vi "Arm State Machine.vi"(1 "Delta Angle":dbl, 2 "Shoulder Control":bool, 3 "Forearm Control":bool, 4 "State":i32) -> (0 "Next State":i32)   [LabVIEW 2017]
uses:
  Robot Global Data.vi
panel:
  in  "Controller Multiplier":dbl=0.5
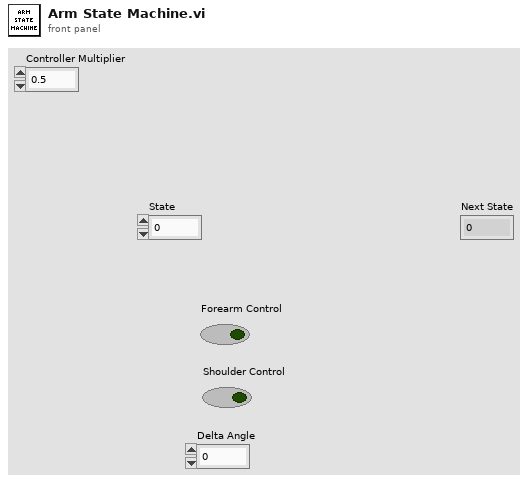
[diagram p1: front panel]
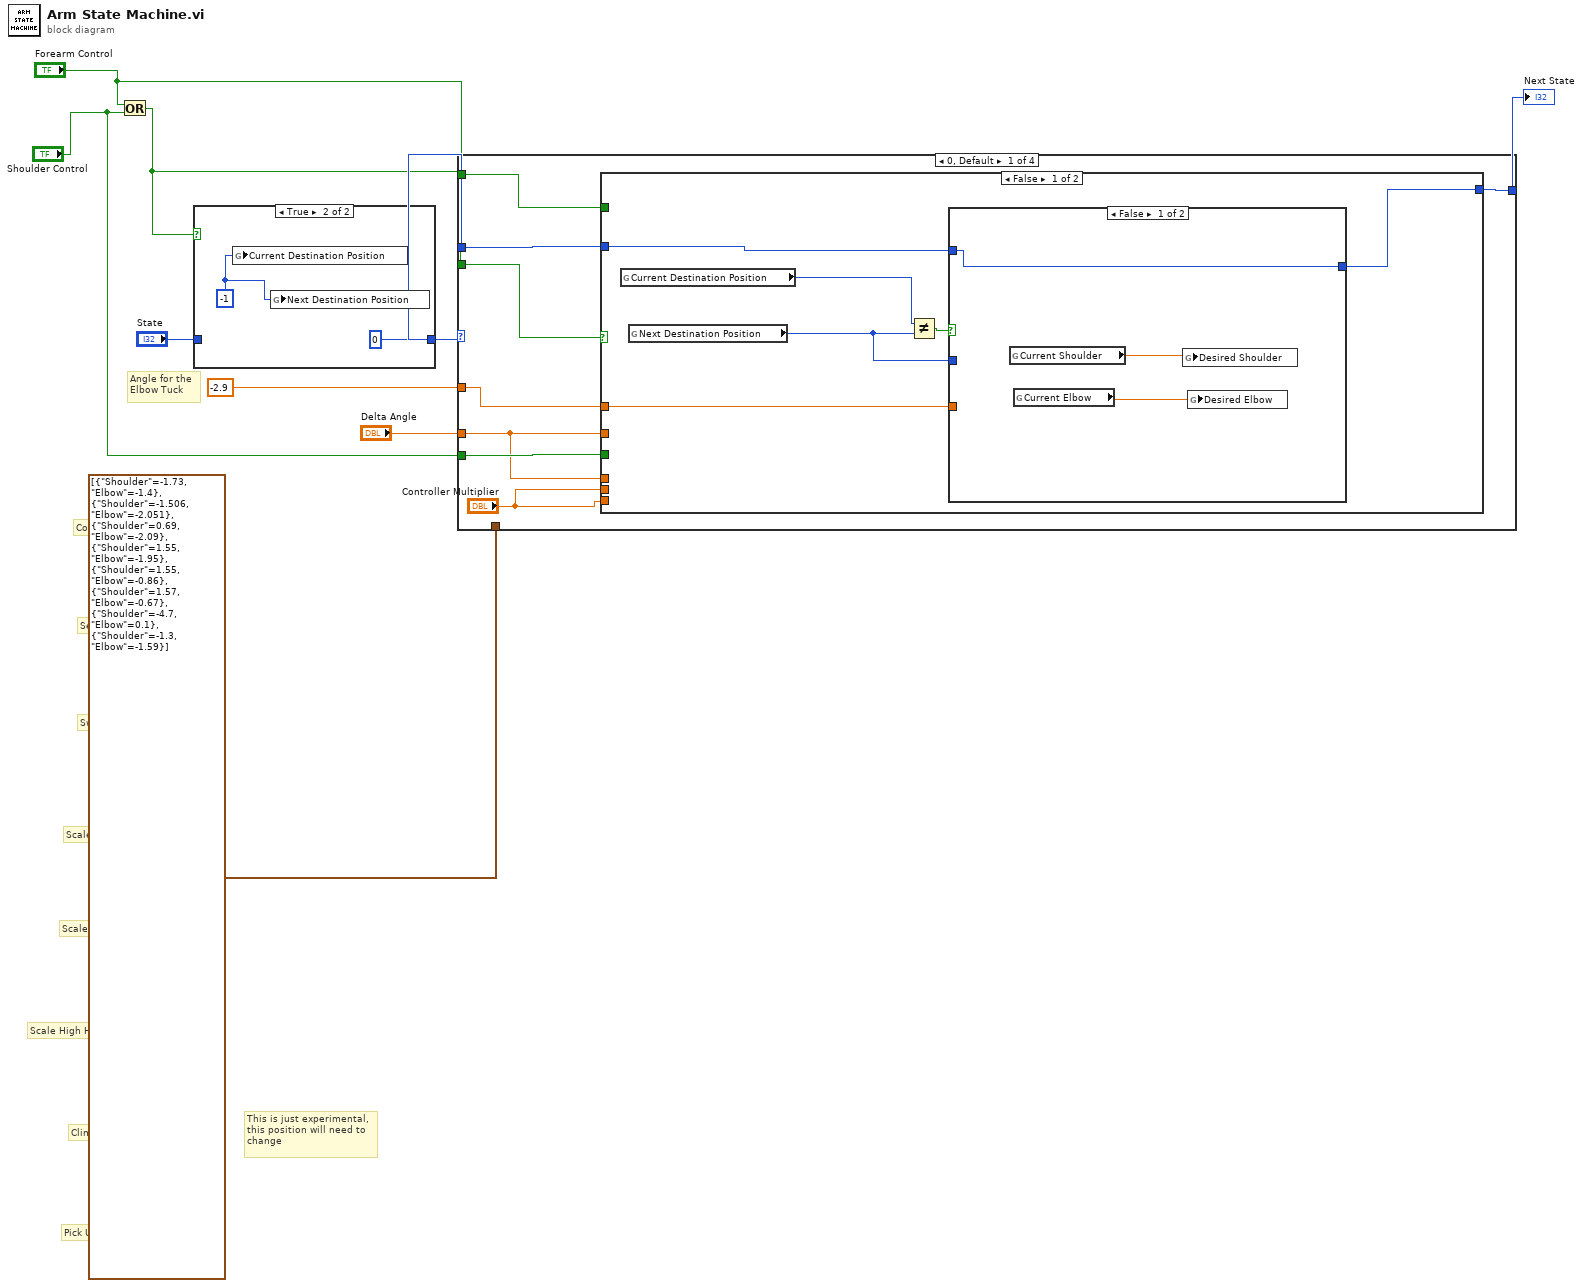
[diagram p0: block diagram]
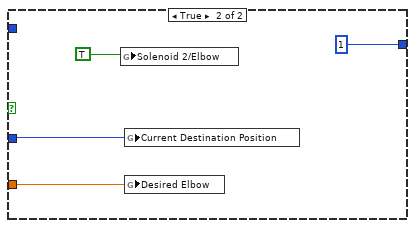
[diagram p3: hidden frame]
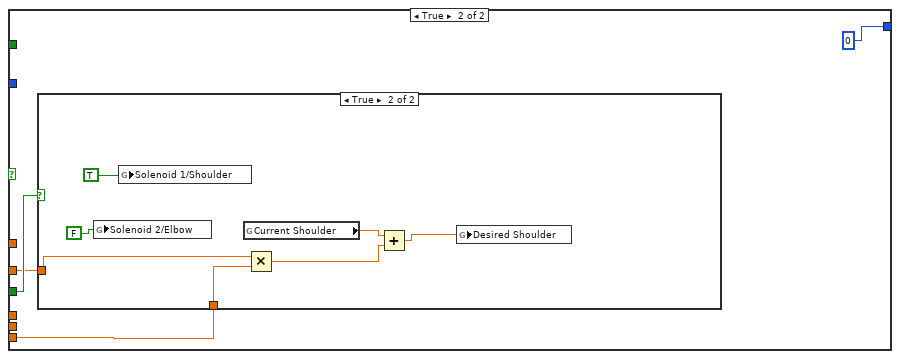
[diagram p4: hidden frame]
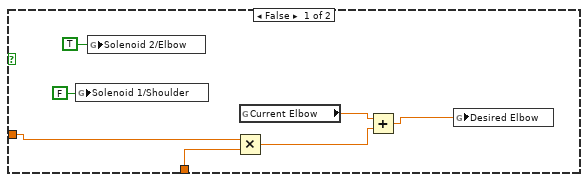
[diagram p5: hidden frame]
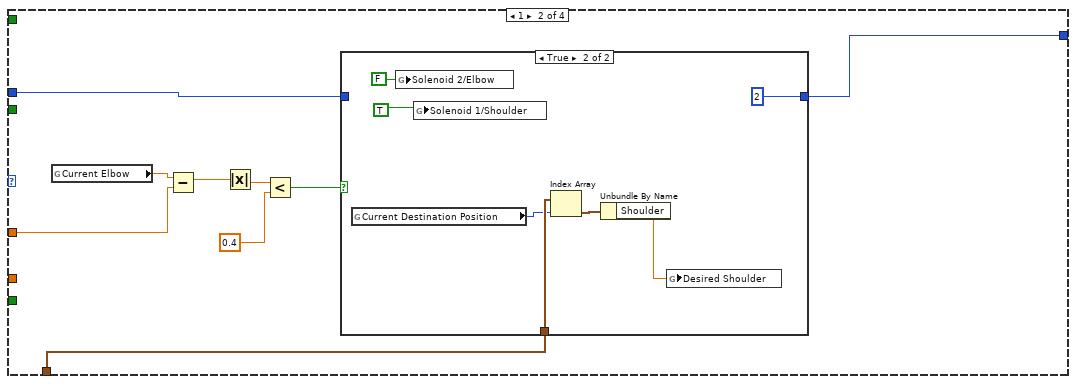
[diagram p6: hidden frame]
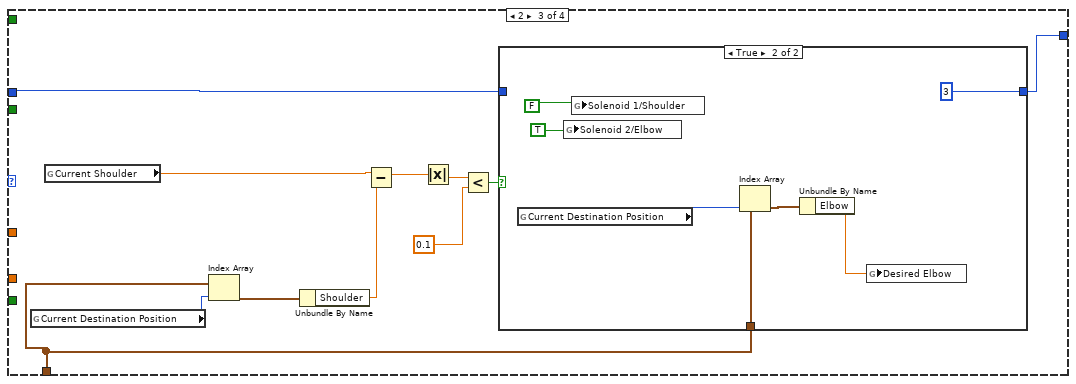
[diagram p8: hidden frame]
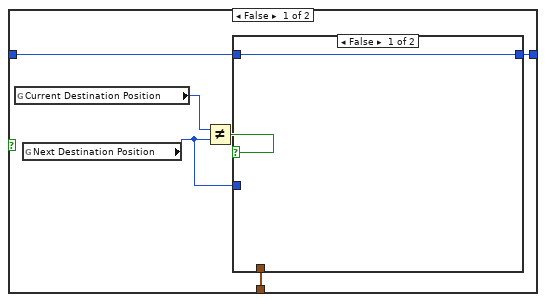
[diagram p9: hidden frame]
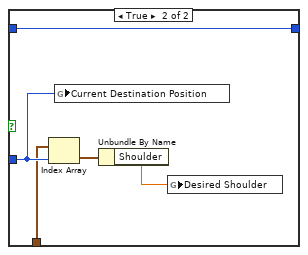
[diagram p10: hidden frame]
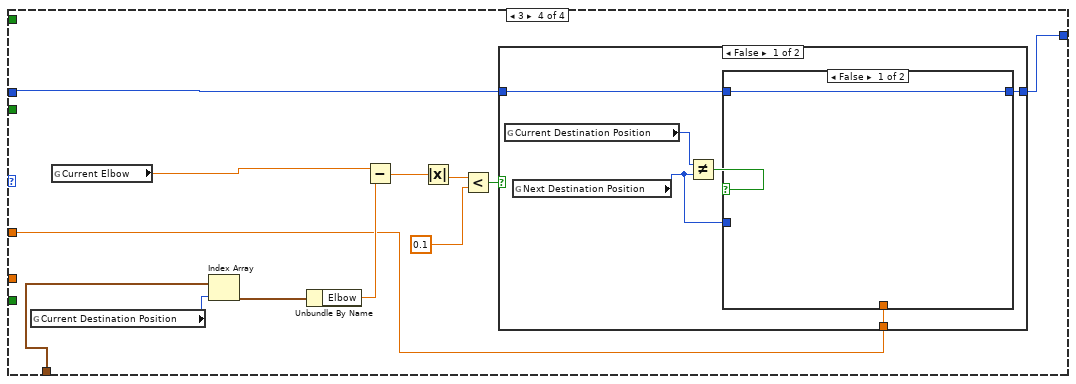
[diagram p11: hidden frame]
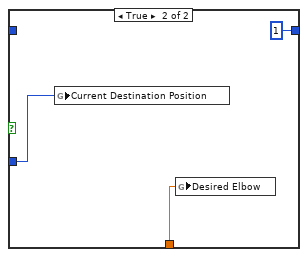
[diagram p12: hidden frame]
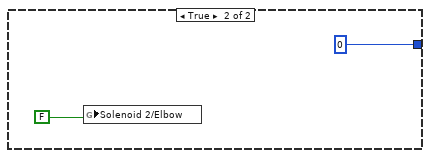
[diagram p13: hidden frame]
diagram:
  # "This is just experimental,\nthis position will need to\nchange"
  # "Pick Up"
  # "Climb"
  # "Scale High High"
  # "Scale High"
  # "Scale Low"
  # "Switch"
  # "Secure"
  # "Collect"
  # "Angle for the\nElbow Tuck"
  n1 = Or(x="Forearm Control", y="Shoulder Control") -> (x .or. y?=w3:bool)
  n2 = case shown="True" w3 {
    tunnel: [w10 0] -> w6
    tunnel: "State" -> [w10 _]
    frame False {
    }
    frame True {
      w11 = -1
      n3 = global write "Robot Global Data.vi" "Current Destination Position"(w11) -> ()
      n4 = global write "Robot Global Data.vi" "Next Destination Position"(w11) -> ()
    }
  }
  n5 = case shown="0, Default" w6 {
    tunnel: w6 -> [w19 w55 w74 w105]
    tunnel: [w20 w54 w73 w104] -> w9
    tunnel: -2.9 -> [w18 w53 _ w99]
    tunnel: cluster{"Shoulder":dbl, "Elbow":dbl}[] [{"Shoulder"=-1.73, "Elbow"=-1.4}, {"Shoulder"=-1.506, "Elbow"=-2.051}, {"Shoulder"=0.69, "Elbow"=-2.09}, {"Shoulder"=1.55, "Elbow"=-1.95}, {"Shoulder"=1.55, "Elbow"=-0.86}, {"Shoulder"=1.57, "Elbow"=-0.67}, {"Shoulder"=-4.7, "Elbow"=0.1}, {"Shoulder"=-1.3, "Elbow"=-1.59}] -> [_ w52 w71 w102]
    tunnel: "Delta Angle" -> [w13 _ _ _]
    tunnel: w3 -> [w17 _ _ _]
    tunnel: "Shoulder Control" -> [w16 _ _ _]
    tunnel: "Forearm Control" -> [w15 _ _ _]
    frame 0, Default {
      n6 = case shown="False" w17 {
        tunnel: [w23 0] -> w20
        tunnel: w19 -> [w22 _]
        tunnel: w18 -> [w21 _]
        tunnel: w16 -> [_ w37]
        tunnel: w15 -> [_ _]
        tunnel: w13 -> [_ _]
        tunnel: "Controller Multiplier" -> [_ _]
        tunnel: "Controller Multiplier" -> [_ w36]
        tunnel: w13 -> [_ w35]
        frame False {
          n7 = global read "Robot Global Data.vi" "Current Destination Position"() -> (w25:i32)
          n8 = global read "Robot Global Data.vi" "Next Destination Position"() -> (w24:i32)
          n9 = Not Equal?(x=w25, y=w24) -> (x != y?=w26:bool)
          n10 = case shown="False" w26 {
            tunnel: w24 -> [_ w32]
            tunnel: [w29 1] -> w23
            tunnel: w22 -> [w29 _]
            tunnel: w21 -> [_ w30]
            frame False {
              n11 = global read "Robot Global Data.vi" "Current Shoulder"() -> (w28:dbl)
              n12 = global read "Robot Global Data.vi" "Current Elbow"() -> (w27:dbl)
              n13 = global write "Robot Global Data.vi" "Desired Shoulder"(w28) -> ()
              n14 = global write "Robot Global Data.vi" "Desired Elbow"(w27) -> ()
            }
            frame True {
              n15 = global write "Robot Global Data.vi" "Solenoid 2/Elbow"(TRUE) -> ()
              n16 = global write "Robot Global Data.vi" "Current Destination Position"(w32) -> ()
              n17 = global write "Robot Global Data.vi" "Desired Elbow"(w30) -> ()
            }
          }
        }
        frame True {
          n18 = case shown="True" w37 {
            tunnel: w36 -> [w38 w46]
            tunnel: w35 -> [w39 w45]
            frame False {
              n19 = global write "Robot Global Data.vi" "Solenoid 1/Shoulder"(FALSE) -> ()
              n20 = global write "Robot Global Data.vi" "Solenoid 2/Elbow"(TRUE) -> ()
              n21 = Multiply(x=w39, y=w38) -> (x*y=w41:dbl)
              n22 = global read "Robot Global Data.vi" "Current Elbow"() -> (w42:dbl)
              n23 = Add(x=w42, y=w41) -> (x+y=w40:dbl)
              n24 = global write "Robot Global Data.vi" "Desired Elbow"(w40) -> ()
            }
            frame True {
              n25 = global write "Robot Global Data.vi" "Solenoid 2/Elbow"(FALSE) -> ()
              n26 = global write "Robot Global Data.vi" "Solenoid 1/Shoulder"(TRUE) -> ()
              n27 = global read "Robot Global Data.vi" "Current Shoulder"() -> (w47:dbl)
              n28 = Multiply(x=w45, y=w46) -> (x*y=w48:dbl)
              n29 = Add(x=w47, y=w48) -> (x+y=w49:dbl)
              n30 = global write "Robot Global Data.vi" "Desired Shoulder"(w49) -> ()
            }
          }
        }
      }
    }
    frame 1 {
      n31 = global read "Robot Global Data.vi" "Current Elbow"() -> (w59:dbl)
      n32 = Subtract(x=w59, y=w53) -> (x-y=w60:dbl)
      n33 = Absolute Value(x=w60) -> (abs(x)=w58:dbl)
      n34 = Less?(x=w58, y=0.4) -> (x < y?=w56:bool)
      n35 = case shown="True" w56 {
        tunnel: w55 -> [w61 _]
        tunnel: [w61 2 ("State")] -> w54
        tunnel: w52 -> [_ w65]
        frame False {
        }
        frame True {
          n36 = global read "Robot Global Data.vi" "Current Destination Position"() -> (w64:i32)
          n37 = global write "Robot Global Data.vi" "Solenoid 2/Elbow"(FALSE ("Solenoid 2/Elbow")) -> ()
          n38 = global write "Robot Global Data.vi" "Solenoid 1/Shoulder"(TRUE ("Solenoid 2/Elbow")) -> ()
          n39 = Index Array(array=w65, index=w64) -> (element=w63:cluster{"Shoulder":dbl, "Elbow":dbl})
          n40 = Unbundle By Name(w63) -> ("Shoulder"=w62:dbl)
          n41 = global write "Robot Global Data.vi" "Desired Shoulder"(w62) -> ()
        }
      }
    }
    frame 2 {
      n42 = global read "Robot Global Data.vi" "Current Destination Position"() -> (w72:i32)
      n43 = global read "Robot Global Data.vi" "Current Shoulder"() -> (w78:dbl)
      n44 = Index Array(array=w71, index=w72) -> (element=w70:cluster{"Shoulder":dbl, "Elbow":dbl})
      n45 = Unbundle By Name(w70) -> ("Shoulder"=w69:dbl)
      n46 = Subtract(x=w78, y=w69) -> (x-y=w79:dbl)
      n47 = Absolute Value(x=w79) -> (abs(x)=w77:dbl)
      n48 = Less?(x=w77, y=0.1) -> (x < y?=w75:bool)
      n49 = case shown="True" w75 {
        tunnel: w74 -> [w83 _]
        tunnel: [w82 3 ("State")] -> w73
        tunnel: w71 -> [w80 w95]
        frame False {
          n50 = global read "Robot Global Data.vi" "Current Destination Position"() -> (w85:i32)
          n51 = global read "Robot Global Data.vi" "Next Destination Position"() -> (w81:i32)
          n52 = Not Equal?(x=w85, y=w81) -> (x != y?=w84:bool)
          n53 = case shown="False" w84 {
            tunnel: w83 -> [w86 w91]
            tunnel: [w86 w91] -> w82
            tunnel: w81 -> [_ w90]
            tunnel: w80 -> [_ w89]
            frame False {
            }
            frame True {
              n54 = Index Array(array=w89, index=w90) -> (element=w88:cluster{"Shoulder":dbl, "Elbow":dbl})
              n55 = global write "Robot Global Data.vi" "Current Destination Position"(w90) -> ()
              n56 = Unbundle By Name(w88) -> ("Shoulder"=w87:dbl)
              n57 = global write "Robot Global Data.vi" "Desired Shoulder"(w87) -> ()
            }
          }
        }
        frame True {
          n58 = global read "Robot Global Data.vi" "Current Destination Position"() -> (w94:i32)
          n59 = global write "Robot Global Data.vi" "Solenoid 2/Elbow"(TRUE ("Solenoid 2/Elbow")) -> ()
          n60 = global write "Robot Global Data.vi" "Solenoid 1/Shoulder"(FALSE ("Solenoid 2/Elbow")) -> ()
          n61 = Index Array(array=w95, index=w94) -> (element=w93:cluster{"Shoulder":dbl, "Elbow":dbl})
          n62 = Unbundle By Name(w93) -> ("Elbow"=w92:dbl)
          n63 = global write "Robot Global Data.vi" "Desired Elbow"(w92) -> ()
        }
      }
    }
    frame 3 {
      n64 = global read "Robot Global Data.vi" "Current Destination Position"() -> (w103:i32)
      n65 = global read "Robot Global Data.vi" "Current Elbow"() -> (w109:dbl)
      n66 = Index Array(array=w102, index=w103) -> (element=w101:cluster{"Shoulder":dbl, "Elbow":dbl})
      n67 = Unbundle By Name(w101) -> ("Elbow"=w100:dbl)
      n68 = Subtract(x=w109, y=w100) -> (x-y=w110:dbl)
      n69 = Absolute Value(x=w110) -> (abs(x)=w108:dbl)
      n70 = Less?(x=w108, y=0.1) -> (x < y?=w106:bool)
      n71 = case shown="False" w106 {
        tunnel: w105 -> [w114 _]
        tunnel: [w113 0 ("State")] -> w104
        tunnel: w99 -> [w111 _]
        frame False {
          n72 = global read "Robot Global Data.vi" "Current Destination Position"() -> (w116:i32)
          n73 = global read "Robot Global Data.vi" "Next Destination Position"() -> (w112:i32)
          n74 = Not Equal?(x=w116, y=w112) -> (x != y?=w115:bool)
          n75 = case shown="False" w115 {
            tunnel: w114 -> [w117 _]
            tunnel: [w117 1 ("State")] -> w113
            tunnel: w112 -> [_ w120]
            tunnel: w111 -> [_ w119]
            frame False {
            }
            frame True {
              n76 = global write "Robot Global Data.vi" "Current Destination Position"(w120) -> ()
              n77 = global write "Robot Global Data.vi" "Desired Elbow"(w119) -> ()
            }
          }
        }
        frame True {
          n78 = global write "Robot Global Data.vi" "Solenoid 2/Elbow"(FALSE) -> ()
        }
      }
    }
  }
  "Next State" <- w9
